vi "Bind Terminal Value.vi"(4 "Ignore Past Updates? (F)":bool, 6 "Value Changes Only? (T)":bool=TRUE, 8 "error in (no error)":errorcluster, 9 "Datum Name (\"\"=Use Control Label)":string, 10 "Ctl Refnum":refnum<vi>, 11 "IViewable in":refnum<class "IViewable.lvclass">) -> (0 "error out":errorcluster, 3 "IViewable out":refnum<class "IViewable.lvclass">)   [LabVIEW 2020, in "IViewable.lvlib" / "IViewable.lvclass"]
doc: "Bind the value of a control terminal (control or indicator) to a publication."
uses:
  <vilib>/gpm_packages/@cs/mva-viewable/Source/IViewable/IViewable/IViewable.lvclass
  C:/Program Files/National Instruments/LabVIEW 2020/vi.lib/ActorFramework/Actor/Actor.lvclass
  <vilib>/ActorFramework/Actor/Actor.lvclass/Actor.ctl
  <vilib>/ActorFramework/Message Enqueuer/Message Enqueuer.lvclass/Message Enqueuer.ctl
  <vilib>/gpm_packages/@cs/mva-core/Source/SubscriptionPolicy/BasicSubscription/BasicSubscription.lvclass/BasicSubscription.ctl
  <vilib>/gpm_packages/@cs/mva-core/Source/SubscriptionPolicy/ValueChangeSubscription/ValueChangeSubscription.lvclass/ValueChangeSubscription.ctl
  <vilib>/gpm_packages/@cs/mva-core/Source/IMediator/SubscriptionRequest/SubscriptionRequest.lvclass/SubscriptionRequest.ctl
  <vilib>/gpm_packages/@cs/mva-core/Source/IObserver/IObserver Messages/Subscribe Msg/Subscribe Msg.lvclass/Subscribe Msg.ctl
  <vilib>/ActorFramework/Message Enqueuer/Enqueue.vi
  <vilib>/ActorFramework/Message Enqueuer/Init from Existing Queue.vi
  <vilib>/gpm_packages/@cs/mva-core/Source/SubscriptionPolicy/BasicSubscription/BasicSubscription.lvclass
  C:/Program Files/National Instruments/LabVIEW 2020/vi.lib/gpm_packages/@cs/mva-core/Source/IMediator/ISubscriptionPolicy/ISubscriptionPolicy.lvclass
  <vilib>/gpm_packages/@cs/mva-core/Source/SubscriptionPolicy/ValueChangeSubscription/ValueChangeSubscription.lvclass
  <vilib>/gpm_packages/@cs/transport/Source/Concrete/TerminalValueBinding/TerminalValueBinding.lvclass
  C:/Program Files/National Instruments/LabVIEW 2020/vi.lib/gpm_packages/@cs/transport/Source/ITransport/ITransport.lvclass
  <vilib>/gpm_packages/@cs/mva-core/Source/IObserver/IObserver Messages/Subscribe Msg/Subscribe Msg.lvclass
  C:/Program Files/National Instruments/LabVIEW 2020/vi.lib/ActorFramework/Message/Message.lvclass
  <vilib>/Utility/error.llb/Error Cluster From Error Code.vi
  <vilib>/ActorFramework/Message Priority Queue/Priority Enqueue.vi
  <vilib>/gpm_packages/@cs/mva-core/Source/IMediator/SubscriptionRequest/SubscriptionRequest.lvclass
  <vilib>/ActorFramework/Message Enqueuer/Message Enqueuer.lvclass
  <vilib>/ActorFramework/Actor/Actor.lvclass
  <vilib>/gpm_packages/@cs/mva-core/Source/IMediator/ISubscriptionPolicy/ISubscriptionPolicy.lvclass
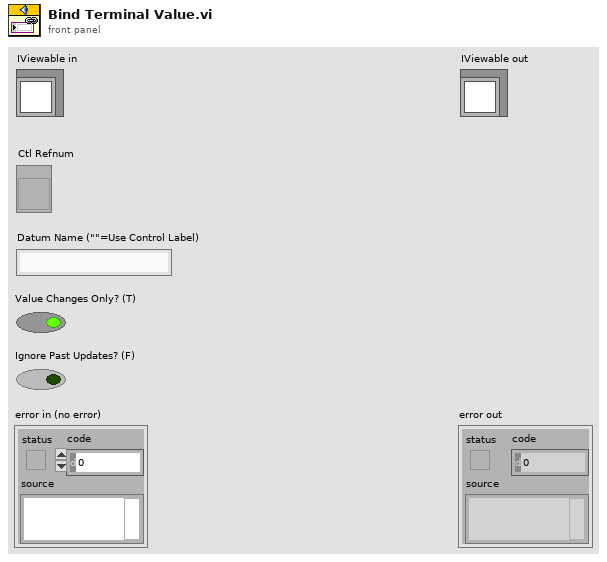
[diagram p1: front panel]
types:
  T1 = typedef "IMediator.lvlib/ISubscriptionPolicy.lvclass/ISubscriptionPolicy Reference.ctl" = refnum<data-value>
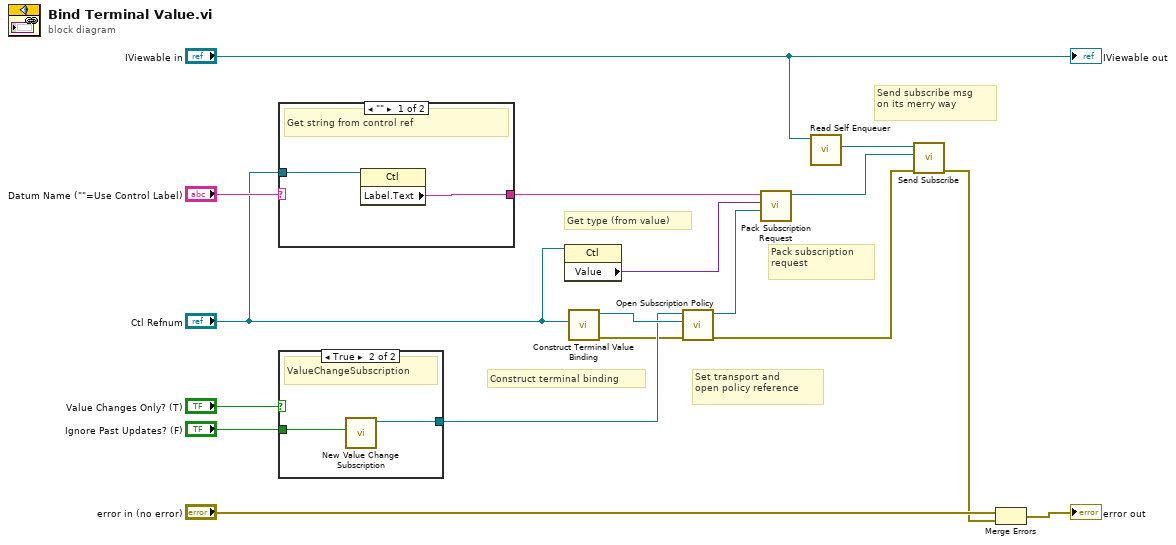
[diagram p0: block diagram]
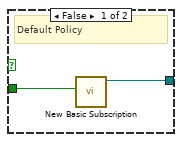
[diagram p2: hidden frame]
diagram:
  # "Set transport and\nopen policy reference"
  # "Send subscribe msg\non its merry way"
  # "Pack subscription\nrequest"
  # "Get type (from value)"
  # "Construct terminal binding"
  n1 = case shown="\"\"" "Datum Name (\"\"=Use Control Label)" {
    selector: "Datum Name (\"\"=Use Control Label)" -> [_ w20]
    tunnel: [w18 w20] -> w9
    tunnel: "Ctl Refnum" -> [w19 _]
    frame "" {
      # "Get string from control ref"
      n2 = property class="Ctl"(reference=w19) -> ("Label.Text"=w18:string)  [unwired: 1 in, 2 out]
    }
    frame Default {
      # "Use string wired to input terminal"
    }
  }
  n3 = case shown="True" "Value Changes Only? (T)" {
    tunnel: "Ignore Past Updates? (F)" -> [w21 w24]
    tunnel: [w22 w23] -> w5
    frame False {
      # "Default Policy"
      n4 = call <vilib>:"New Basic Subscription.vi"("Ignore Past Updates? (F)"=w21) -> ("BasicSubscription Out"=w22:refnum<class "BasicSubscription.lvclass">)  [unwired: 10 in]
    }
    frame True {
      # "ValueChangeSubscription"
      n5 = call <vilib>:"New Value Change Subscription.vi"("Ignore Past Updates? (F)"=w24) -> ("ValueChangeSubscription Out"=w23:refnum<class "ValueChangeSubscription.lvclass">)  [unwired: 10 in]
    }
  }
  n6 = property class="Ctl"(reference="Ctl Refnum") -> ("Value"=w16:variant)  [unwired: 1 in, 2 out]
  n7 = call <vilib>:"Construct Terminal Value Binding.vi"("Ctl Refnum"="Ctl Refnum") -> ("error out"=w1:errorcluster, "TerminalValueBinding Out"=w7:refnum<class "TerminalValueBinding.lvclass">)  [unwired: 9 in]
  n8 = call <vilib>:"Open Subscription Policy.vi"("error in (no error)"=w1, "Transport"=w7, "SubscriptionPolicy"=w5) -> ("error out"=w2:errorcluster, "Subscription Policy"=w3:T1)  [unwired: 7 in]
  n9 = call <vilib>:"Pack Subscription Request.vi"("Subscription Policy"=w3, "Type"=w16, "Datum Name"=w9) -> ("SubscriptionRequest"=w13:refnum<class "SubscriptionRequest.lvclass">)  [unwired: 7 in, 1 out]
  n10 = call <vilib>:"Read Self Enqueuer.vi"("Actor"="IViewable in") -> ("Self Enqueuer"=w14:refnum<class "Message Enqueuer.lvclass">)  [unwired: 10 in]
  n11 = call <vilib>:"Send Subscribe.vi"("error in (no error)"=w2, "SubscriptionRequest"=w13, "Message Enqueuer"=w14) -> ("error out"=w11:errorcluster)  [unwired: 7 in, 1 out]
  n12 = Merge Errors("error in (no error)", w11) -> (→"error out":errorcluster)
  "IViewable out" <- "IViewable in"
